vi "M9290A Set Freq and Acquire Peak.vi"(6 "Route Names":string[](array[string]), 7 "Cal?":bool, 8 "error in (no error)":errorcluster, 9 "Span(Hz)":dbl=26500000000.0, 10 "Center Frequency(Hz)":u64=13250000000, 11 "VISA resource name":refnum<visa-resource-name>) -> (0 "error out":errorcluster, 1 "Amplitude (Cal)":dbl, 2 "Frequency":dbl format="%#_6f", 3 "VISA out":refnum<visa-resource-name>, 4 "FDelta":dbl)   [LabVIEW 2014]
uses:
  Agilent MXA Series/Configure Frequency (Center Span).vi
  Agilent MXA Series.lvlib
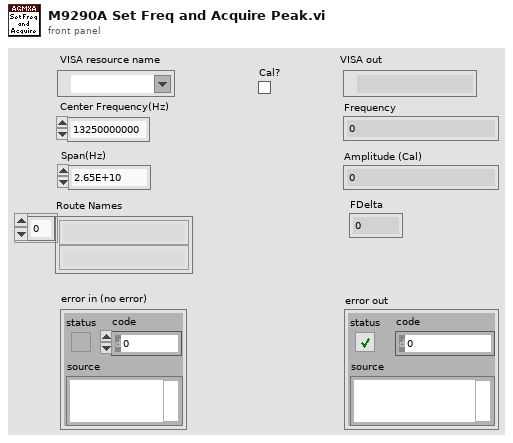
[diagram p1: front panel]
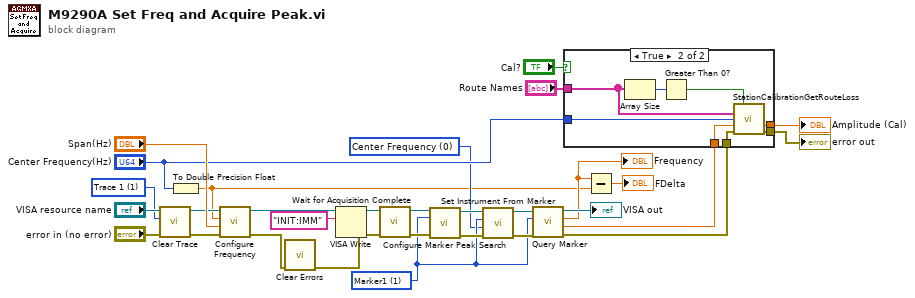
[diagram p0: block diagram]
diagram:
  w3 = 1 items=["Trace 1"=1, "Trace 2"=2, "Trace 3"=3, "Trace 4"=4, "Trace 5"=5, "Trace 6"=6, "All"=7] ("Trace  (1: Trace 1)")
  w8 = 0 items=["Center Frequency", "Center Frequency Step", "Start Frequency", "Stop Frequency", "Delta Span", "Delta Center Frequency", "Reference Level"] ("Instrument Setting (0: Center Frequency)")
  w9 = 1 items=["Marker1"=1, "Marker2"=2, "Marker3"=3, "Marker4"=4, "Marker5"=5, "Marker6"=6, "Marker7"=7, "Marker8"=8, "Marker9"=9, "Marker10"=10, "Marker11"=11, "Marker12"=12] ("Active Marker (1: Marker1)")
  n1 = call "Clear Trace.vi"("error in (no error)"="error in (no error)", "Trace  (1: Trace 1)"=w3, "VISA resource name"="VISA resource name") -> ("error out"=w5:errorcluster, "VISA resource name out"=w4:refnum<visa-resource-name>)  [unwired: 7 in]
  n2 = To Double Precision Float(number="Center Frequency(Hz)") -> (double precision float=w2:dbl)
  n3 = call-poly "Configure Frequency.vi"("error in (no error)"=w5, "Span (2.65E+10 Hz)"="Span(Hz)", "Center Frequency (1.325E+10 Hz)"=w2, "VISA resource name"=w4) -> ("error out"=w15:errorcluster, "VISA resource name out"=w17:refnum<visa-resource-name>)  [unwired: 6 in]
  n4 = call "Clear Errors.vi"("error in (no error)"=w15) -> ("error out"=w14:errorcluster)  [unwired: 5 in, 1 out]
  n5 = VISA Write(VISA resource name=w17, write buffer="INIT:IMM" ("format string"), error in (no error)=w14) -> (VISA resource name out=w29:refnum<visa-resource-name>, error out=w28:errorcluster)  [unwired: 1 out]
  n6 = call "Wait for Acquisition Complete.vi"("error in (no error)"=w28, "VISA resource name"=w29) -> ("error out"=w19:errorcluster, "VISA resource name out"=w18:refnum<visa-resource-name>)  [unwired: 8 in]
  n7 = call "Configure Marker Peak Search.vi"("VISA resource name"=w18, "Active Marker (1: Marker1)"=w9, "error in (no error)"=w19) -> ("VISA resource name out"=w12:refnum<visa-resource-name>, "error out"=w13:errorcluster)  [unwired: 11 in]
  n8 = call "Set Instrument From Marker.vi"("error in (no error)"=w13, "Instrument Setting (0: Center Frequency)"=w8, "Active Marker (1: Marker1)"=w9, "VISA resource name"=w12) -> ("error out"=w11:errorcluster, "VISA resource name out"=w10:refnum<visa-resource-name>)  [unwired: 6 in]
  n9 = call "Query Marker.vi"("error in (no error)"=w11, "Active Marker (1: Marker1)"=w9, "VISA resource name"=w10) -> ("error out"=w25:errorcluster, "Marker Amplitude"=w26:dbl, "Marker Position"=w22:dbl, "VISA resource name out"=→"VISA out":refnum<visa-resource-name>)  [unwired: 5 in]
  "Frequency" <- w22
  n10 = case shown="True" "Cal?" {
    tunnel: [w32 w41] -> w27
    tunnel: w26 -> [w32 w40]
    tunnel: w25 -> [w33 w39]
    tunnel: [w33 w38] -> w24
    tunnel: "Route Names" -> [_ w37]
    tunnel: "Center Frequency(Hz)" -> [_ w35]
    frame False {
    }
    frame True {
      n11 = Array Size(array=w37) -> (size(s)=w36:i32)
      n12 = Greater Than 0?(x=w36) -> (x > 0?=w34:bool)
      n13 = call "StationCalibrationGetRouteLoss.vi"("Calibration Enabled"=w34, "Route Names"=w37, "Frequency"=w35, "Power Level"=w40, "error in (no error)"=w39) -> ("Adjusted Power Level"=w41:dbl, "error out"=w38:errorcluster)  [unwired: 7 in, 2 out]
    }
  }
  "error out" <- w24
  "Amplitude (Cal)" <- w27
  n14 = Subtract(x=w22, y=w2) -> (x-y=→"FDelta":dbl)
